vi "Responce Parse.vi"(11 "Responce":string) -> (1 "Payload":string, 2 "Command":string, 3 "Address":u8, 5 "OK":bool, 7 "Checksum OK":bool)   [LabVIEW 2016, in "Samwontech TEMP2xxx.lvlib"]
uses:
  <instrlib>/Samwontech TEMP2xxx/Samwontech TEMP2xxx.lvlib
panel:
  out "Probe: Calculated \nSUM (byte)":u8 format="%.0x"
  out "Probe: Responce SUM":string
  out "Probe: Responce without SUM":string
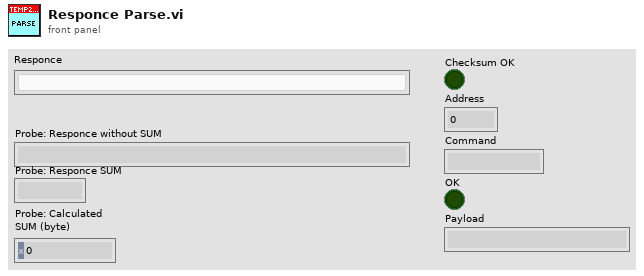
[diagram p1: front panel]
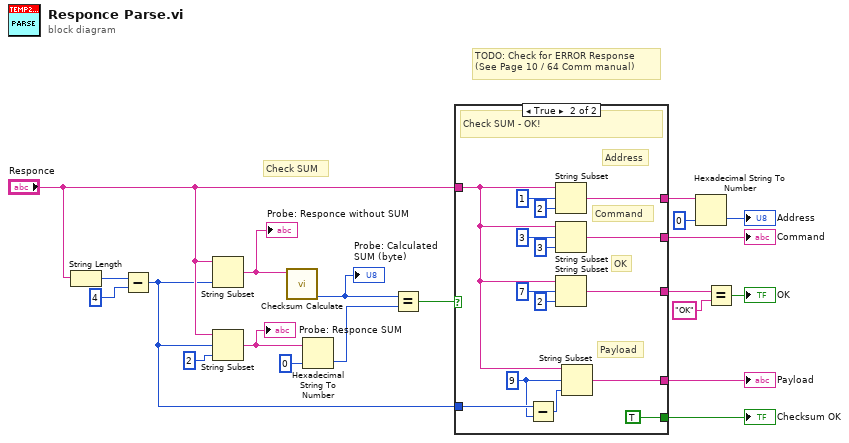
[diagram p0: block diagram]
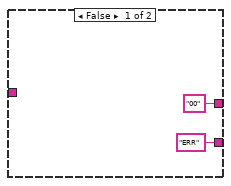
[diagram p2: hidden frame]
diagram:
  # "Check SUM"
  # "TODO: Check for ERROR Response \n(See Page 10 / 64 Comm manual)"
  n1 = String Length(string="Responce") -> (length=w20:i32)
  n2 = Subtract(x=w20, y=4) -> (x-y=w6:i32)
  n3 = String Subset(string="Responce", length (rest)=w6) -> (substring=w17:string)  [unwired: 1 in]
  "Probe: Responce without SUM" <- w17
  n4 = String Subset(string="Responce", offset (0)=w6, length (rest)=2 ("length (rest)")) -> (substring=w16:string)
  "Probe: Responce SUM" <- w16
  n5 = call <instrlib>:"Checksum Calculate.vi"("Command in"=w17) -> ("Checksum (byte)"=w15:u8)  [unwired: 7 in, 3 out]
  "Probe: Calculated \nSUM (byte)" <- w15
  n6 = Hexadecimal String To Number(string=w16, default (0uL)=u8 0) -> (number=w14:u8)  [unwired: 1 in, 1 out]
  n7 = Equal?(x=w15, y=w14) -> (x = y?=w13:bool)
  n8 = case shown="True" w13 {
    tunnel: "Responce" -> [_ w24]
    tunnel: ["ERR" ("Responce") w25] -> w11
    tunnel: ["00" ("Responce") w33] -> w8
    tunnel: [_ w32] -> w5
    tunnel: w6 -> [_ w31]
    tunnel: [_ TRUE] -> w4
    tunnel: [_ w23] -> w3
    frame False {
    }
    frame True {
      w30 = 9 ("length (rest)")
      # "OK"
      # "Payload"
      # "Command"
      # "Address"
      # "Check SUM - OK!"
      n9 = Subtract(x=w31, y=w30) -> (x-y=w29:i32)
      n10 = String Subset(string=w24, offset (0)=1 ("length (rest)"), length (rest)=2 ("length (rest)")) -> (substring=w33:string)
      n11 = String Subset(string=w24, offset (0)=3 ("length (rest)"), length (rest)=3 ("length (rest)")) -> (substring=w25:string)
      n12 = String Subset(string=w24, offset (0)=7 ("length (rest)"), length (rest)=2 ("length (rest)")) -> (substring=w23:string)
      n13 = String Subset(string=w24, offset (0)=w30, length (rest)=w29) -> (substring=w32:string)
    }
  }
  "Command" <- w11
  "Payload" <- w5
  "Checksum OK" <- w4
  n14 = Hexadecimal String To Number(string=w8, default (0uL)=u8 0) -> (number=→"Address":u8)  [unwired: 1 in, 1 out]
  n15 = Equal?(x=w3, y="OK") -> (x = y?=→"OK":bool)
